vi "Clear Current Value Table.vi"(8 "error in (no error)":errorcluster) -> (0 "error out":errorcluster)   [LabVIEW 2020, in "Current Value Table(Rebuild).lvlib"]
doc: "This VI reinitializes all CVT items and clears old data from memory."
uses:
  FGVs/Group Memory Methods.ctl
  FGVs/Tag Memory Methods.ctl
  Memory Block.vi
  DataTypes/Array of String_Memory Block.vi
  DataTypes/Array of Boolean_Memory Block.vi
  DataTypes/Array of Single_Memory Block.vi
  DataTypes/Array of Double_Memory Block.vi
  DataTypes/Array of I8_Memory Block.vi
  DataTypes/Array of I16_Memory Block.vi
  DataTypes/Array of I32_Memory Block.vi
  DataTypes/Array of I64_Memory Block.vi
  DataTypes/Array of U64_Memory Block.vi
  DataTypes/Array of U32_Memory Block.vi
  DataTypes/Array of U16_Memory Block.vi
  DataTypes/Array of U8_Memory Block.vi
  DataTypes/Boolean_Memory Block.vi
  DataTypes/String_Memory Block.vi
  DataTypes/U8_Memory Block.vi
  DataTypes/U16_Memory Block.vi
  DataTypes/U32_Memory Block.vi
  DataTypes/U64_Memory Block.vi
  DataTypes/I8_Memory Block.vi
  DataTypes/I16_Memory Block.vi
  DataTypes/I32_Memory Block.vi
  DataTypes/I64_Memory Block.vi
  DataTypes/Single_Memory Block.vi
  DataTypes/Double_Memory Block.vi
  FGVs/CVT Globals.vi
  Current Value Table(Rebuild).lvlib
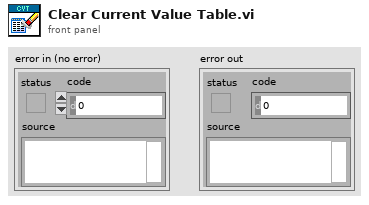
[diagram p1: front panel]
types:
  T1 = typedef "Current Value Table(Rebuild).lvlib/Group Memory Methods.ctl" = enum16{"Clear", "Read Indices in Group", "List Groups", "List Tags by Type", "List Tags", "Delete Group", "Check Group Existence", "Create Group"}
  T2 = typedef "Current Value Table(Rebuild).lvlib/Tag Memory Methods.ctl" = enum16{"Clear", "Read Tag Index", "Read Tag Indices", "Generate Group", "Add Tag", "Overwrite Tag", "Read Description", "Get Stored Tags", "Write Description"}
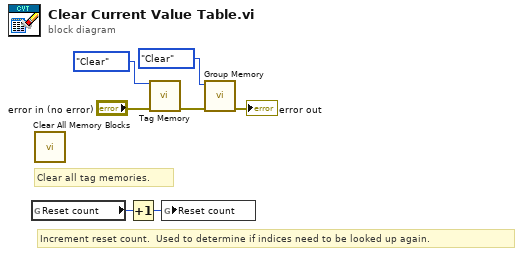
[diagram p0: block diagram]
diagram:
  # "Increment reset count.  Used to determine if indices need to be looked up again."
  # "Clear all tag memories."
  n1 = global read "CVT Globals.vi" "Reset count"() -> (w2:u32)
  n2 = call "Clear All Memory Blocks.vi"() -> ()  [unwired: 12 in]
  n3 = Increment(x=w2) -> (x+1=w1:u32)
  n4 = call "Tag Memory.vi"("Method"=Tag_Memory_Methods."Clear", "error in (no error)"="error in (no error)") -> ("error out"=w5:errorcluster)  [unwired: 8 in, 5 out]
  n5 = global write "CVT Globals.vi" "Reset count"(w1) -> ()
  n6 = call "Group Memory.vi"("error in (no error)"=w5, "Method"=Group_Memory_Methods."Clear") -> ("error out"=→"error out":errorcluster)  [unwired: 6 in, 3 out]
